vi "FGV_Enable-Disable SkipList.vi"(7 "FGV_Enable-Disable SkipList_Commands":T1=enum."Initialize", 8 "Error In":errorcluster, 11 "Skip control name IN":string) -> (0 "Error Out":errorcluster, 3 "Skip array OUT":string[](array[string]))   [LabVIEW 2012]
doc: "SciScan 1.2 160622\nThis FGV stores and updates the GFG variables that need to be skipped during an enable/disable operation. This is to avoid global Enable/Disable actions affecting the Enabled/Disabled behaviour implemented in specific modules"
uses:
  FGV_Enable-Disable SkipList_Commands.ctl
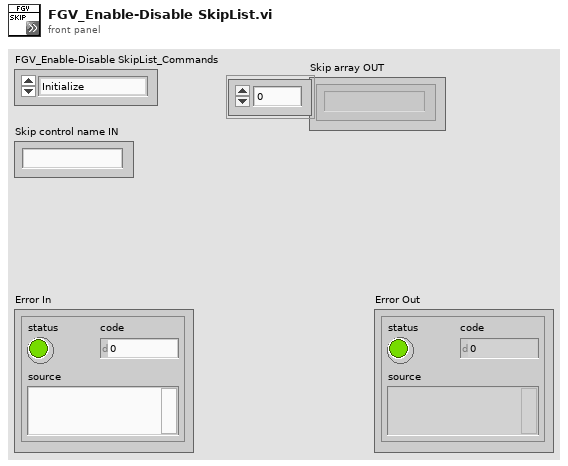
[diagram p1: front panel]
types:
  T1 = typedef "FGV_Enable-Disable SkipList_Commands.ctl" = enum16{"Get List", "Initialize", "Update List"}
  T2 = enum8{"Enabled", "Disabled", "Disabled and Grayed Out"}
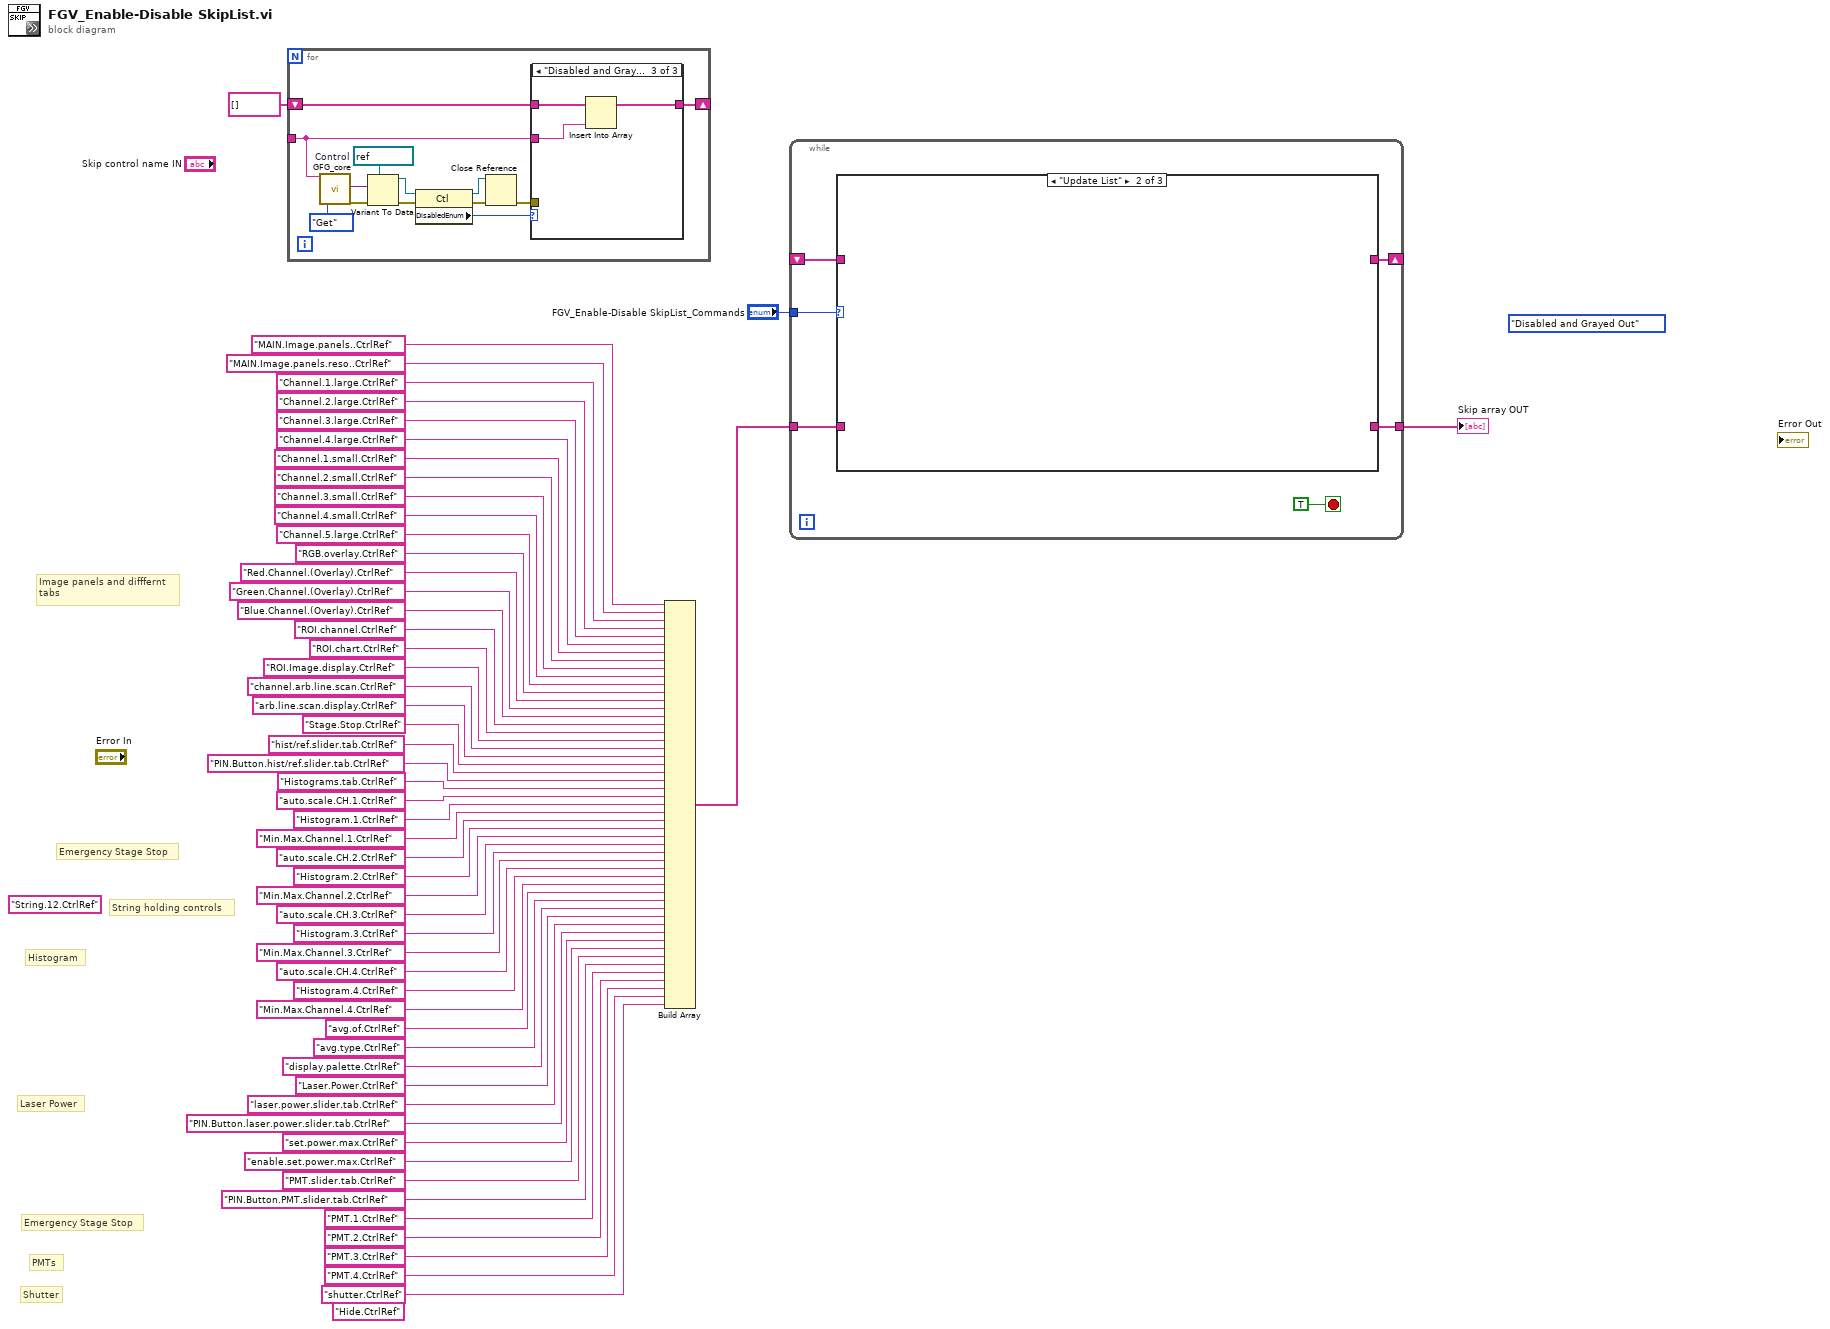
[diagram p0: block diagram]
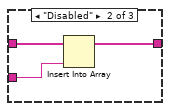
[diagram p3: hidden frame]
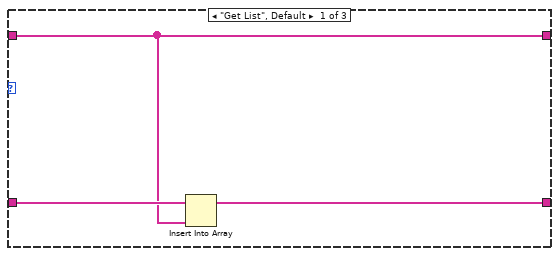
[diagram p4: hidden frame]
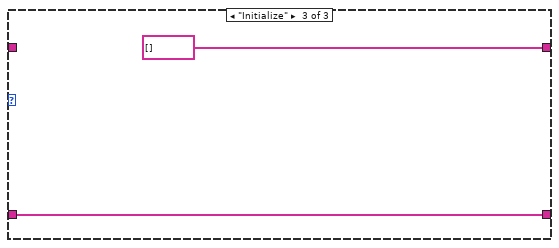
[diagram p5: hidden frame]
diagram:
  (unwired) T2."Disabled and Grayed Out" ("Disabled")
  (unwired) "Hide.CtrlRef"
  (unwired) "String.12.CtrlRef"
  # "Image panels and difffernt\ntabs"
  # "Histogram"
  # "Laser Power"
  # "PMTs"
  # "Shutter"
  # "Emergency Stage Stop"
  # "String holding controls"
  # "Emergency Stage Stop"
  n1 = for {
    tunnel: [w58] -> w2
    shift-right: [w59] -> w3
    shift-left: string[] [] ("All Variable Names Out") -> [w60]
    w68 = refnum<vi> refnum  # Control
    n2 = call "GFG_core.vi"("Variable Name in"=w58, "Action"=enum16{"Init", "Set", "Get", "Clear"}."Get") -> ("Variant Out"=w66:variant, "error out"=w67:errorcluster)  [unwired: 11 in, 5 out]
    n3 = Variant To Data(error in=w67, type=w68, Variant=w66) -> (data=w64:refnum<vi>, error out=w63:errorcluster)
    n4 = property class="Ctl"(reference=w64, error in=w63) -> (reference out=w69:refnum<vi>, error out=w70:errorcluster, "DisabledEnum"=w62:T2)
    n5 = Close Reference(reference=w69, error in (no error)=w70) -> (error out=w61:errorcluster)
    n6 = case shown="\"Disabled and Grayed Out\"" w62 {
      tunnel: w61 -> [_ _ _]
      tunnel: w60 -> [w71 w74 w77]
      tunnel: [w71 w73 w76] -> w59
      tunnel: w58 -> [_ w72 w75]
      frame "Enabled", Default {
      }
      frame "Disabled" {
        n7 = Insert Into Array(array=w74, new element=w72) -> (w73:string[])  [unwired: 1 in]
      }
      frame "Disabled and Grayed Out" {
        n8 = Insert Into Array(array=w77, new element=w75) -> (w76:string[])  [unwired: 1 in]
      }
    }
  }
  n9 = Build Array("MAIN.Image.panels..CtrlRef", "MAIN.Image.panels.reso..CtrlRef", "Channel.1.large.CtrlRef", "Channel.2.large.CtrlRef", "Channel.3.large.CtrlRef", "Channel.4.large.CtrlRef", "Channel.1.small.CtrlRef", "Channel.2.small.CtrlRef", "Channel.3.small.CtrlRef", "Channel.4.small.CtrlRef", "Channel.5.large.CtrlRef", "RGB.overlay.CtrlRef", "Red.Channel.(Overlay).CtrlRef", "Green.Channel.(Overlay).CtrlRef", "Blue.Channel.(Overlay).CtrlRef", "ROI.channel.CtrlRef", "ROI.chart.CtrlRef", "ROI.Image.display.CtrlRef", "channel.arb.line.scan.CtrlRef", "arb.line.scan.display.CtrlRef", "Stage.Stop.CtrlRef", "hist/ref.slider.tab.CtrlRef", "PIN.Button.hist/ref.slider.tab.CtrlRef", "Histograms.tab.CtrlRef", "auto.scale.CH.1.CtrlRef", "Histogram.1.CtrlRef", "Min.Max.Channel.1.CtrlRef", "auto.scale.CH.2.CtrlRef", "Histogram.2.CtrlRef", "Min.Max.Channel.2.CtrlRef", "auto.scale.CH.3.CtrlRef", "Histogram.3.CtrlRef", "Min.Max.Channel.3.CtrlRef", "auto.scale.CH.4.CtrlRef", "Histogram.4.CtrlRef", "Min.Max.Channel.4.CtrlRef", "avg.of.CtrlRef", "avg.type.CtrlRef", "display.palette.CtrlRef", "Laser.Power.CtrlRef", "laser.power.slider.tab.CtrlRef", "PIN.Button.laser.power.slider.tab.CtrlRef", "set.power.max.CtrlRef", "enable.set.power.max.CtrlRef", "PMT.slider.tab.CtrlRef", "PIN.Button.PMT.slider.tab.CtrlRef", "PMT.1.CtrlRef", "PMT.2.CtrlRef", "PMT.3.CtrlRef", "PMT.4.CtrlRef", "shutter.CtrlRef") -> (w5:string[])
  n10 = while {
    tunnel: "FGV_Enable-Disable SkipList_Commands" -> [w83]
    tunnel: w5 -> [w81]
    shift-right: [w80] -> _
    shift-left: _ -> [w79]
    tunnel: [w78] -> w4
    stop <- TRUE stop-if-true
    n11 = case shown="\"Update List\"" w83 {
      tunnel: w81 -> [w86 _ w87]
      tunnel: [w85 _ string[] []] -> w80
      tunnel: w79 -> [w85 _ _]
      tunnel: [w84 _ w87] -> w78
      frame "Get List", Default {
        n12 = Insert Into Array(array=w86, new element=w85) -> (w84:string[])  [unwired: 1 in]
      }
      frame "Update List" {
      }
      frame "Initialize" {
      }
    }
  }
  "Skip array OUT" <- w4
